vi "Warning Queu Updater.vi"(8 "Current Warning Num":i32, 9 "Existing Num Array":i32[](array[numeric]), 10 "Warning Array In":string[](array[string])) -> (2 "Updated Existing Array":i32[](array[numeric]), 3 "Warning Array Out":string[](array[string]))   [LabVIEW 2013]
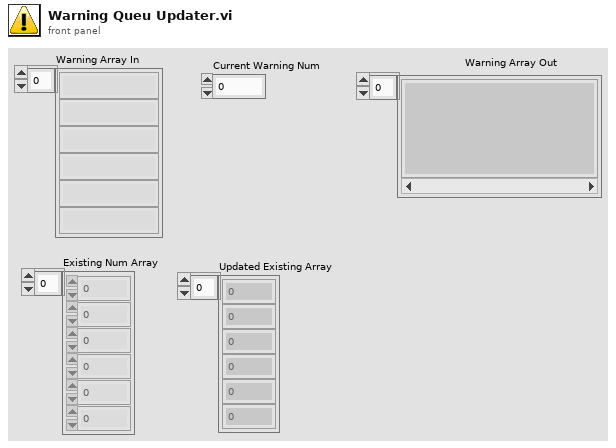
[diagram p1: front panel]
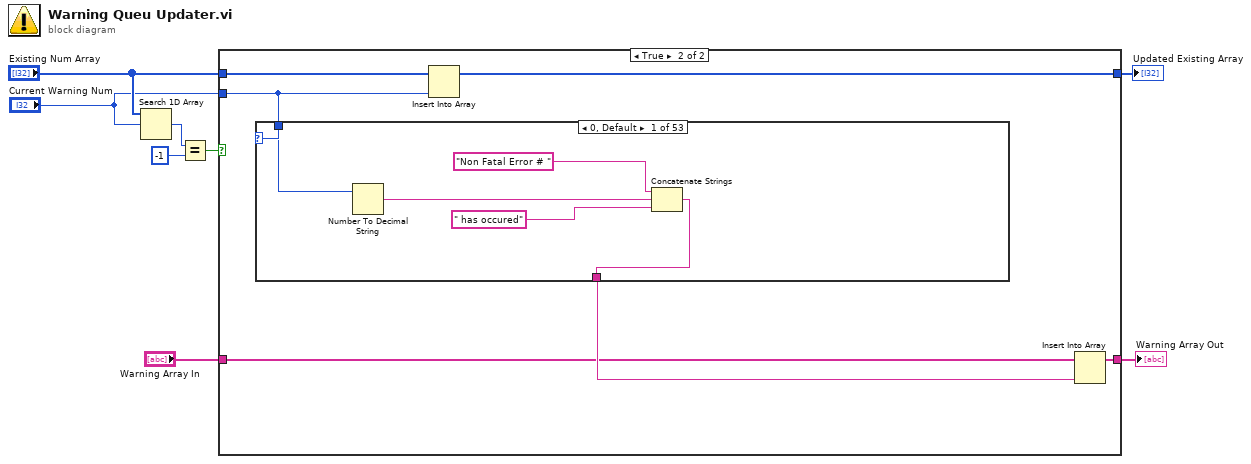
[diagram p0: block diagram]
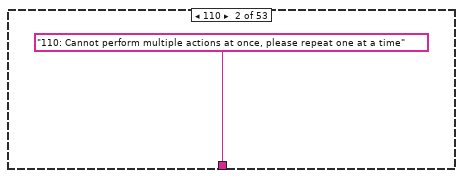
[diagram p3: hidden frame]
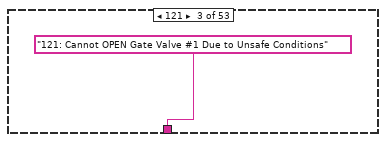
[diagram p4: hidden frame]
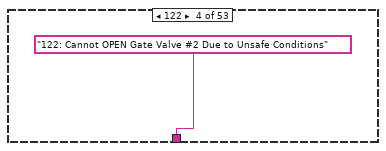
[diagram p5: hidden frame]
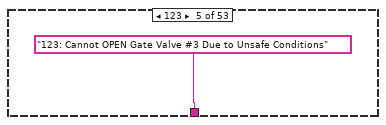
[diagram p6: hidden frame]
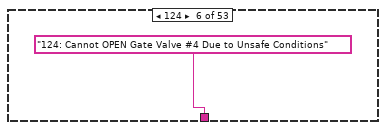
[diagram p7: hidden frame]
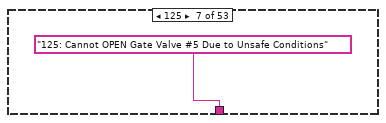
[diagram p8: hidden frame]
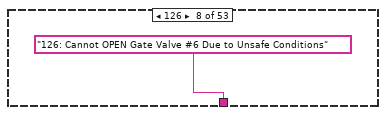
[diagram p9: hidden frame]
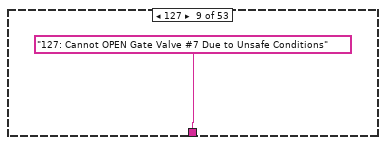
[diagram p10: hidden frame]
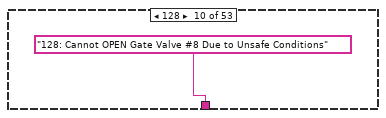
[diagram p11: hidden frame]
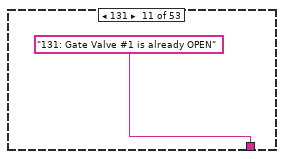
[diagram p12: hidden frame]
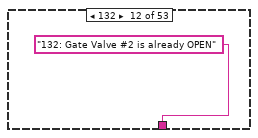
[diagram p13: hidden frame]
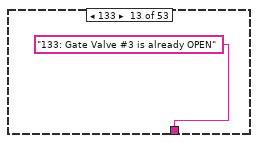
[diagram p14: hidden frame]
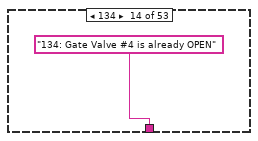
[diagram p15: hidden frame]
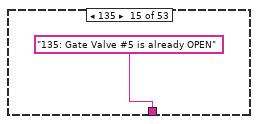
[diagram p16: hidden frame]
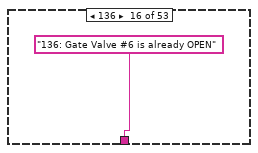
[diagram p17: hidden frame]
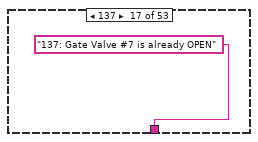
[diagram p18: hidden frame]
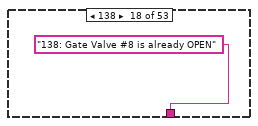
[diagram p19: hidden frame]
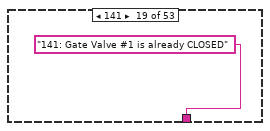
[diagram p20: hidden frame]
diagram:
  n1 = Search 1D Array(1D array="Existing Num Array", element="Current Warning Num") -> (index of element=w2:i32)  [unwired: 1 in]
  n2 = Equal?(x=w2, y=-1) -> (x = y?=w5:bool)
  n3 = case shown="True" w5 {
    tunnel: [w9 w15] -> w8
    tunnel: "Warning Array In" -> [w9 w14]
    tunnel: "Existing Num Array" -> [w10 w13]
    tunnel: [w10 w12] -> w3
    tunnel: "Current Warning Num" -> [_ w11]
    frame False {
    }
    frame True {
      n4 = case shown="0, Default" w11 {
        tunnel: [w17 "110: Cannot perform multiple actions at once, please repeat one at a time" "121: Cannot OPEN Gate Valve #1 Due to Unsafe Conditions" "122: Cannot OPEN Gate Valve #2 Due to Unsafe Conditions" "123: Cannot OPEN Gate Valve #3 Due to Unsafe Conditions" "124: Cannot OPEN Gate Valve #4 Due to Unsafe Conditions" "125: Cannot OPEN Gate Valve #5 Due to Unsafe Conditions" "126: Cannot OPEN Gate Valve #6 Due to Unsafe Conditions" "127: Cannot OPEN Gate Valve #7 Due to Unsafe Conditions" "128: Cannot OPEN Gate Valve #8 Due to Unsafe Conditions" "131: Gate Valve #1 is already OPEN" "132: Gate Valve #2 is already OPEN" "133: Gate Valve #3 is already OPEN" "134: Gate Valve #4 is already OPEN" "135: Gate Valve #5 is already OPEN" "136: Gate Valve #6 is already OPEN" "137: Gate Valve #7 is already OPEN" "138: Gate Valve #8 is already OPEN" "141: Gate Valve #1 is already CLOSED" "142: Gate Valve #2 is already CLOSED" "143: Gate Valve #3 is already CLOSED" "144: Gate Valve #4 is already CLOSED" "145: Gate Valve #5 is already CLOSED" "146: Gate Valve #6 is already CLOSED" "147: Gate Valve #7 is already CLOSED" "148: Gate Valve #8 is already CLOSED" "150: Tried to OPEN or CLOSE a Gate Valve that is in MANUAL OVERIDE MODE" "160: Tried to OPEN/CLOSE a Cryopump Gate Valve, this funtionality is temporarily disabled, use manual override mode" "211: Automatically CLOSED Gate Valve #1 Due to unsafe conditions" "212 Automatically CLOSED Gate Valve #2 Due to unsafe conditions" "213: Automatically CLOSED Gate Valve #3 Due to unsafe conditions" "214: Automatically CLOSED Gate Valve #4 Due to unsafe conditions" "215: Automatically CLOSED Gate Valve #5 Due to unsafe conditions" "216: Automatically CLOSED Gate Valve #6 Due to unsafe conditions" "217: Automatically CLOSED Gate Valve #7 Due to unsafe conditions" "218: Automatically CLOSED Gate Valve #8 Due to unsafe conditions" "221: Sent a signal to OPEN a Gate Valve #1 and didnt see response in 100ms, please check hardware connections" "222: Sent a signal to OPEN a Gate Valve #2 and didnt see response in 100ms, please check hardware connections" "223: Sent a signal to OPEN a Gate Valve #3 and didnt see response in 100ms, please check hardware connections" "224: Sent a signal to OPEN a Gate Valve #4 and didnt see response in 100ms, please check hardware connections" "226: Sent a signal to OPEN a Gate Valve #6 and didnt see response in 100ms, please check hardware connections" "226: Sent a signal to OPEN a Gate Valve #6 and didnt see response in 100ms, please check hardware connections" "227: Sent a signal to OPEN a Gate Valve #7 and didnt see response in 100ms, please check hardware connections" "228: Sent a signal to OPEN a Gate Valve #8 and didnt see response in 100ms, please check hardware connections" "231: Sent a signal to CLOSE a Gate Valve #1 and didnt see response in 100ms, please check hardware connections" "232: Sent a signal to CLOSE a Gate Valve #2 and didnt see response in 100ms, please check hardware connections" "233: Sent a signal to CLOSE a Gate Valve #3 and didnt see response in 100ms, please check hardware connections" "234: Sent a signal to CLOSE a Gate Valve #4 and didnt see response in 100ms, please check hardware connections" "235: Sent a signal to CLOSE a Gate Valve #5 and didnt see response in 100ms, please check hardware connections" "236: Sent a signal to CLOSE a Gate Valve #6 and didnt see response in 100ms, please check hardware connections" "237: Sent a signal to CLOSE a Gate Valve #7 and didnt see response in 100ms, please check hardware connections" "238: Sent a signal to CLOSE a Gate Valve #8 and didnt see response in 100ms, please check hardware connections" "Testing warning case."] -> w16
        tunnel: w11 -> [w20 _ _ _ _ _ _ _ _ _ _ _ _ _ _ _ _ _ _ _ _ _ _ _ _ _ _ _ _ _ _ _ _ _ _ _ _ _ _ _ _ _ _ _ _ _ _ _ _ _ _ _ _]
        frame 0, Default {
          n5 = Number To Decimal String(number=w20) -> (decimal integer string=w19:string)  [unwired: 1 in]
          n6 = Concatenate Strings("Non Fatal Error # ", w19, " has occured" ("string")) -> (w17:string)
        }
        frame 110 {
        }
        frame 121 {
        }
        frame 122 {
        }
        frame 123 {
        }
        frame 124 {
        }
        frame 125 {
        }
        frame 126 {
        }
        frame 127 {
        }
        frame 128 {
        }
        frame 131 {
        }
        frame 132 {
        }
        frame 133 {
        }
        frame 134 {
        }
        frame 135 {
        }
        frame 136 {
        }
        frame 137 {
        }
        frame 138 {
        }
        frame 141 {
        }
        frame 142 {
        }
        frame 143 {
        }
        frame 144 {
        }
        frame 145 {
        }
        frame 146 {
        }
        frame 147 {
        }
        frame 148 {
        }
        frame 150 {
        }
        frame 160 {
        }
        frame 211 {
        }
        frame 212 {
        }
        frame 213 {
        }
        frame 214 {
        }
        frame 215 {
        }
        frame 216 {
        }
        frame 217 {
        }
        frame 218 {
        }
        frame 221 {
        }
        frame 222 {
        }
        frame 223 {
        }
        frame 224 {
        }
        frame 225 {
        }
        frame 226 {
        }
        frame 227 {
        }
        frame 228 {
        }
        frame 231 {
        }
        frame 232 {
        }
        frame 233 {
        }
        frame 234 {
        }
        frame 235 {
        }
        frame 236 {
        }
        frame 237 {
        }
        frame 238 {
        }
        frame 999 {
        }
      }
      n7 = Insert Into Array(array=w13, new element=w11) -> (w12:i32[])  [unwired: 1 in]
      n8 = Insert Into Array(array=w14, new element=w16) -> (w15:string[])  [unwired: 1 in]
    }
  }
  "Warning Array Out" <- w8
  "Updated Existing Array" <- w3
